vi "读取数据转DBL.vi"(1 "读取数据":string) -> (0 "DBL":dbl[][](array[numeric]))   [LabVIEW 2020]
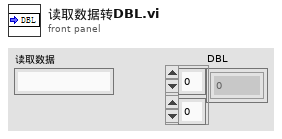
[diagram p1: front panel]
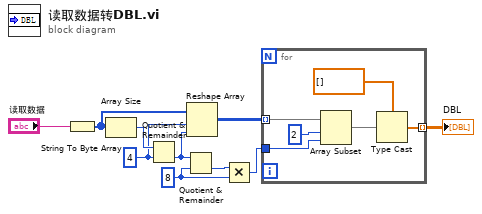
[diagram p0: block diagram]
diagram:
  w2 = 8 ("y")
  w6 = 4 ("维数大小")
  n1 = String To Byte Array(string="读取数据") -> (unsigned byte array=w8:u8[])
  n2 = Array Size(array=w8) -> (size(s)=w7:i32)
  n3 = Quotient & Remainder(x=w7, y=w6) -> (floor(x/y)=w4:i32)  [unwired: 1 out]
  n4 = Quotient & Remainder(x=w4, y=w2) -> (floor(x/y)=w3:i32)  [unwired: 1 out]
  n5 = Reshape Array(w8, w6, w4) -> (w5:u8[][])
  n6 = Multiply(x=w3, y=w2) -> (x*y=w1:i32)
  n7 = for {
    tunnel: [w16] -> w10 mode=indexing
    tunnel: w5 -> [w14] mode=indexing
    tunnel: w1 -> [w12]
    n8 = Array Subset(array=w14, index=2 ("索引"), length=w12) -> (w11:u8[])
    n9 = Type Cast(type=dbl[] [] ("*(类型 *) &x"), x=w11) -> (*(type *) &x=w16:dbl[])
  }
  "DBL" <- w10
